vi "QWTB Algorithms Configurator Panel.vi"(8 "error in":errorcluster, 11 "session out":T1={"adc"={"niScope"={"channel cfg"=[], "sessions"=[], "multi cards"=FALSE, "channels"=0, "type"=enum."n/a", "memory [B/chn]"=0, "ext. clock [Hz]"=0.0, "samples count"=0, "use streaming"=FALSE, "proc setup"={"packet size [smpl]"=0, "current timeout [s]"=0.0, "blk2blk timeout [s]"=0.0, "event time"=timestamp(0 s since 1904-01-01), "temp sampl T [s]"=0.0, "data queue"=refnum, "stop notifier"=refnum, "proc ref"=refnum}, "sample width [B]"=0, "ranges [V]"=[], "trigger setup"={"coupling"=1, "level [V]"=0.0, "slope"=0, "mode"=enum."Immediate", "pre-trigger [%]"=0.0}, "fs [Hz]"=0.0, "bitres [bit]"=0, "clock source"=enum."VAL_NO_SOURCE"}, "3458A"={"channels"=[], "sync unit"={"VISA"="", "type"=enum."Picotest U6200A"}, "awg unit"={"type"=enum."Agilent 331xxA to 332xxA", "VISA"="", "enable 10MHz ref"=FALSE, "cmi ckd2"={"VISA"="", "clock source"=enum."Auto", "manual ref clk"=FALSE, "ref clock [Hz]"=0.0, "div mode"=enum."Set divisor directly"}, "cmi sync v3"={"VISA"="", "baud rate [bd/s]"=115200, "source"=enum."Auto", "hv range"=enum."1kV", "fsrc is fixed"=FALSE, "fsrc [Hz]"=10000000.0, "freq integ [s]"=1.0, "freq filter"=5, "trig level"=enum."TTL 5V", "chn1 mode"=enum."Source divider", "chn1 level"=enum."Positive 5V", "chn2 mode"=enum."Source divider", "chn2 level"=enum."Positive 5V", "chn2 div"=1, "chn3 mode"=enum."Chn 1 Active", "chn3 level"=enum."Positive 5V", "chn1 div entry"=enum."Calculate nearest divisor from measured fx", "chn1 dev limit [%]"=1.0, "chn1 check dev"=FALSE}, "trigger"={"source"=enum."Immediate", "slope"=enum."POS", "coupling"=enum."DC", "level [V]"=0.0, "hysteresis [V]"=0.0, "pre-trigger [%]"=0.0}, "HMF2500 cfg"={"Baud Rate"=9600, "Parity"=0, "Data Bits"=8, "Flow Control"=4}}, "sync mode"=enum."MASTER-SLAVE, MASTER clocked by TIMER", "streaming mode"=FALSE, "idn mode"=enum."Auto", "sampling mode"=enum."DCV", "sample memory [B]"=0, "proc setup"={"channel id"=0, "packet size [smpl]"=0, "current timeout [s]"=0.0, "blk2blk timeout [s]"=0.0, "event time"=timestamp(0 s since 1904-01-01), "stop notifier"=refnum, "data queues"=[], "proc refs"=[], "bus semaphore"=refnum}, "sample size [B]"=0, "sample count"=0, "aux data"={"channel id"=0, "valid?"=[], "gain [V]"=[], "timestamp [s]"=[], "Ts [s]"=0.0, "abs timestamp"=timestamp(0 s since 1904-01-01), "t [deg C]"=[], "multiplex timestamp [s]"=-1.0, "only multiplex?"=FALSE, "multiplex smpl offset"=0, "overflow?"=FALSE}, "ranges [V]"=[], "aperture [s]"=0.0, "LEVEL trigger"={"edge"=enum."POS", "level [V]"=0.0, "coupling"=enum."DC"}, "trigger mode"=enum."AUTO", "measure temp.?"=FALSE, "disp mesages"=[], "shared bus?"=FALSE, "disable display?"=FALSE, "aper mode"=enum."Manual", "aper rules"=[], "multiplex"={"cycles"=0, "delay [s]"=0.0, "enabled"=FALSE, "overhead [s]"=1.0, "tot smpls"=0, "sub-rec"=0, "overhead [%]"=0.0, "emulated"=FALSE}, "F8588 lpf"=enum."Off", "F8588 pll"=enum."Off", "F8588 couple"=enum."DC, auto", "fs"={"freq mode"=enum."fs or Ts", "fs [Hz]"=0.0, "fref [Hz]"=0.0, "mul"=0.0, "div"=0.0}, "fs mode"=enum."fs or Ts", "init timestamp"=timestamp(0 s since 1904-01-01), "last report timestamp"=timestamp(0 s since 1904-01-01)}, "dsdll"={"dsdll"={"dsdll path"=path "", "dsdll handle"=[], "output devices"=[], "capture devices"=[]}, "channels"=0, "device id"=0, "channel idns"=[], "proc setup"={"packet size [smpl]"=0, "current timeout [s]"=0.0, "blk2blk timeout [s]"=0.0, "event time"=timestamp(0 s since 1904-01-01), "data queue"=refnum, "stop notifier"=refnum, "proc ref"=refnum}, "samples count"=0, "fs [Hz]"=0.0}, "type"=enum."niScope", "channel idn str"=[], "aux instr idn str"=[], "modified?"=FALSE, "simadc"={"channels"=[], "range [V]"=0.0, "Ts step [s]"=0.0, "time [s]"=0.0, "fs [Hz]"=0.0, "count"=0, "smpl offset"=0, "set count"=0, "bit res"=0}, "force rst?"=FALSE, "exit mode"=enum."Immediate reset", "exit dly"=0.0, "exit tmr"=timestamp(0 s since 1904-01-01), "busy?"=FALSE, "accessed?"=FALSE, "multiplex"={"Type"=enum."Dummy", "gen com ssn"={"visa"="", "primary"=enum."None", "secondary"=enum."None", "channels"=[]}, "delay before [s]"=0.0, "delay post [s]"=0.0, "sequence"=[], "enabled"=FALSE, "ref timestamp [s]"=0.0, "idn string"="", "dev niScope"="", "niScope idx"=0, "QPMX ssn"={"visa"="", "switch mode"=enum."Switched by TWM", "sequence"=[], "timing delays"=[], "polarity"=enum."Positive", "ss delay (s)"=2.0, "internal timer (s)"=1.0, "Last loaded sequence file"=path "", "startup delay (s)"=2.0}, "VISA mux ssn"={"VISA"="", "paths"=[], "idn command"="", "serial cfg"={"Baud rate"=9600, "Data bits"=8, "Parity"=0, "Stop bits"=10, "Flow control"=0, "End Mode Read"=enum."None", "End Mode Write"=enum."None", "Term character"=0, "Term enable"=FALSE}}}, "keysight dso"={"VISA"="", "channels"=[], "bw limit [Hz]"=0.0, "resolution"=enum."Basic", "trig noise reject"=enum."Normal", "N"=0, "trigger config"={"trigger source"=enum."Immediate", "trigger slope"=enum."Negative", "level [V]"=0.0, "hysteresis [V]"=0.001, "pre-trig [%]"=50}, "fs [Hz]"=0.0, "timeout stop"=timestamp(0 s since 1904-01-01), "waiting for opc"=FALSE, "fetch offset [smpl]"=0, "abs timestamp"=timestamp(0 s since 1904-01-01), "ranges [V]"=[], "decimation"=1.0, "ext ref"=FALSE, "emulate aperture"=FALSE, "model"=enum."DSO91304"}, "cdaq"={"mclk [Hz]"=12800000.0, "ADC task"="", "mclk reference"="", "fs [Hz]"=50000.0, "queue adc cmd"=refnum, "queue adc data"=refnum, "adc proc ref"=refnum, "channels"=[], "last channels"=[], "timeout"=timestamp(0 s since 1904-01-01), "N"=1000, "mclk mode"=enum."Free running", "ext mclk source"=""}, "ignore overload"=FALSE, "ADS127L21"={"VISA"="", "chn list"=[], "record size"=0, "phys. channels"=0, "adc fifo size"=0, "channels"=[], "ext refclk?"=FALSE, "fs [Hz]"=0.0, "ext refclk [Hz]"=0.0, "meas refclk [Hz]"=0.0, "EXTOUT mode"=enum."ADCCLK", "EXTOUT polarity"=enum."NORM", "EXTOUT divisor"=0}}, "sequence"=[], "sequence setup"={"group setups"=[], "rec count"=0, "range mode"=enum."Keep defaults", "fs mode"=enum."Frequency", "rng even"=0.0, "rng odd"=0.0, "folder"=path "", "name base"="", "meas id"=0, "settle [s]"=0.0, "comment"="", "avg count"=0, "fs-abs-fr fr"=0.0, "fs-abs-fr fs"=0.0, "fs-div fr"=0.0, "fs-div div"=0.0, "fs-mn fr"=0.0, "fs-mn mul"=0.0, "fs-mn div"=0.0, "fs-rat fr"=0.0, "fs-rat rat"=0.0}, "golpi"=refnum, "processing setup"={"mode"=enum."Raw", "call after avgs?"=FALSE, "calculate?"=FALSE, "raw mode"={"command"="", "result mode"=enum."Display console output (only Octave)", "res variable"=""}, "QWTB"={"QWTB path"=path "F:/TWM/octprog/qwtb", "alg filter path"="octprog\\qwtb_list.info", "alg ids"=[], "alg parameters"=[], "parsed parameters"=[], "selected alg id"="", "selected unc mode"=enum."None", "qwtb mcc"=100, "qwtb timeout"=90, "qwtb covg"=95.0, "qwtb ofs"=0, "qwtb lim data"=0, "multicore"={"jobs folder"=path "", "cores"=0, "max jobs"=0, "mode"=enum."Singlecore"}, "unc once?"=FALSE, "qwtb tstemp"=enum."Enabled (default)", "octave reset"=FALSE, "exec mode"=enum."Single-core"}}, "corrections"={"transducers"={"channels"=[], "last path"=path "", "root path"=path ""}, "digitizer"={"last path"=path "", "channel paths"=[], "channel idns"=[], "correction name"="", "channel names"=[], "folders to copy"=[], "channel valid"=[], "correction path"=path "", "correction rel path"="", "rel folders to copy"=[], "root path"=path ""}}, "assist cfg"={"P"=0, "Q"=0, "rel shift"=0.0, "ref freq"=0.0, "min fs"=0.0, "max fs tol"=0.0, "min int"=0.0, "max int"=0.0, "max err"=0.0, "max timeout"=0.0}} {"corrections"."transducers"."channels"."Phase index" min=1 step=1; "adc"."ADS127L21"."channels"."Channel" min=1 max=8 step=1; "adc"."ADS127L21"."channels"."Range [Vpk]" items=["±1.65V", "±2V"]; "adc"."cdaq"."last channels"."Channel id" min=0 step=1; "adc"."cdaq"."channels"."Channel id" min=0 step=1; "adc"."keysight dso"."decimation" min=1.0; "adc"."keysight dso"."bw limit [Hz]" format="%#_6p"; "adc"."keysight dso"."channels"."Offset [V]" format="%#_6p"; "adc"."keysight dso"."channels"."Range [Vpk]" min=0.0 format="%#_6p"; "adc"."keysight dso"."channels"."Channel" min=1; "adc"."multiplex"."VISA mux ssn"."serial cfg"."Flow control" items=["None", "XON/XOFF", "CTS/RTS", "XON/XOFF + CTS/RTS", "DTR/DSR", "XON/XOFF + DTR/DSR"]; "adc"."multiplex"."VISA mux ssn"."serial cfg"."Stop bits" items=["1 bit"=10, "1.5 bits"=15, "2 bits"=20]; "adc"."multiplex"."VISA mux ssn"."serial cfg"."Parity" items=["None", "Odd", "Even", "Mark", "Space"]; "adc"."multiplex"."VISA mux ssn"."serial cfg"."Data bits" items=["5 bits"=5, "6 bits"=6, "7 bits"=7, "8 bits"=8]; "adc"."multiplex"."VISA mux ssn"."serial cfg"."Baud rate" items=["150 Bd"=150, "300 Bd"=300, "600 Bd"=600, "1200 Bd"=1200, "2400 Bd"=2400, "4800 Bd"=4800, "9600 Bd"=9600, "19.2 kBd"=19200, "38.4 kBd"=38400, "57.6 kBd"=57600, "115.2 kBd"=115200]; "adc"."multiplex"."QPMX ssn"."startup delay (s)" min=0.0 step=1.0; "adc"."multiplex"."QPMX ssn"."internal timer (s)" min=0.0 step=1.0; "adc"."multiplex"."QPMX ssn"."ss delay (s)" min=0.0 step=1.0; "adc"."multiplex"."QPMX ssn"."timing delays" min=1 max=255 step=1; "adc"."3458A"."awg unit"."HMF2500 cfg"."Flow Control" items=["None", "XON/XOFF", "RTS/CTS", "XON/XOFF & RTS/CTS", "DTR/DSR", "XON/XOFF & DTR/DSR"]; "adc"."3458A"."awg unit"."HMF2500 cfg"."Data Bits" items=["7"=7, "8"=8]; "adc"."3458A"."awg unit"."HMF2500 cfg"."Parity" items=["None", "Odd", "Even", "Mark", "Space"]; "adc"."3458A"."awg unit"."HMF2500 cfg"."Baud Rate" items=["300"=300, "600"=600, "1200"=1200, "2400"=2400, "4800"=4800, "9600"=9600, "19200"=19200]; "adc"."3458A"."awg unit"."cmi sync v3"."chn2 div" min=1 max=100000000 step=1; "adc"."3458A"."awg unit"."cmi sync v3"."fsrc [Hz]" format="%_8p"; "adc"."3458A"."channels"."Range [Vpk]" min=0.0; "adc"."niScope"."trigger setup"."pre-trigger [%]" format="%.2f"; "adc"."niScope"."trigger setup"."level [V]" format="%.2f"; "adc"."niScope"."trigger setup"."coupling" items=["AC"=0, "DC"=1, "HF Reject"=3, "LF Reject"=4, "AC Plus HF Reject"=1001]; "adc"."niScope"."channel cfg"."Range [Vpk]" min=0.0; "adc"."niScope"."channel cfg"."Channel" min=0}) -> (0 "error out":errorcluster)   [LabVIEW 2020]
doc: "Configuration panel for QWTB algorithms."
uses:
  Meas Session.ctl
  adc/ADC Session.ctl
  drivers/niScope/niScope Session.ctl
  drivers/niScope/niScope Virtual Channel Config.ctl
  drivers/niScope/niScope Virtual Channel Mode.ctl
  drivers/niScope/niScope Virtual Channel Input Z.ctl
  drivers/niScope/niScope Virtual Channel Coupling.ctl
  drivers/niScope/niScope Type.ctl
  drivers/niScope/niScope Digitizing Process Options.ctl
  drivers/niScope/niScope Data Packet.ctl
  drivers/niScope/niScope Trigger Setup.ctl
  <instrlib>/niScope/Controls/niScope trigger coupling.ctl
  <instrlib>/niScope/Controls/niScope trigger slope.ctl
  drivers/niScope/niScope Reference Clock.ctl
  drivers/DMM/3458A Digitizer Session.ctl
  drivers/DMM/3458A Virtual Channel Config.ctl
  drivers/Counter/Counter Session.ctl
  drivers/Counter/Counter Type.ctl
  drivers/AWG/AWG Session.ctl
  drivers/AWG/AWG Type.ctl
  drivers/AWG/CMI Clock Divider v2/CMI ckd2 Session.ctl
  drivers/AWG/CMI Clock Divider v2/CMI ckd2 Source Mode.ctl
  drivers/AWG/CMI Clock Divider v2/CMI ckd2 Divisor Mode.ctl
  drivers/AWG/CMI Sync V3/CMI Sync V3 session.ctl
  drivers/AWG/CMI Sync V3/Configure/CMI Sync V3 Reference Clock Source.ctl
  drivers/AWG/CMI Sync V3/Configure/CMI Sync V3 HV input Range.ctl
  drivers/AWG/CMI Sync V3/Configure/CMI Sync V3 Trigger Input Level.ctl
  drivers/AWG/CMI Sync V3/Configure/CMI Sync V3 Channel 1 Mode.ctl
  drivers/AWG/CMI Sync V3/Configure/CMI Sync V3 Channel Output Levels.ctl
  drivers/AWG/CMI Sync V3/Configure/CMI Sync V3 Channel 2 Mode.ctl
  drivers/AWG/CMI Sync V3/Configure/CMI Sync V3 Channel 3 Mode.ctl
  drivers/AWG/CMI Sync V3/Configure/CMI Sync V3 Channel 1 Divisor Entry Mode.ctl
  adc/ADC Trig Config.ctl
  adc/ADC Trig Mode Source.ctl
  adc/ADC Trig Slope.ctl
  adc/ADC Trig Coupling.ctl
  drivers/AWG/RaS HMF2500/HMF2500 Config.ctl
  drivers/DMM/3458A Sync Mode.ctl
  drivers/DMM/3458A Idn Mode.ctl
  drivers/DMM/3458A Digitizing Low Levels/Configure/Sampling Mode.ctl
  drivers/DMM/3458A Digitizing Process Options.ctl
  drivers/DMM/3458A Data Packet.ctl
  drivers/DMM/3458A Aux Record Data.ctl
  drivers/DMM/3458A Digitizing Low Levels/Configure/Level Setup.ctl
  drivers/DMM/3458A Digitizing Low Levels/Configure/First Sample Trigger.ctl
  drivers/DMM/3458A Aperture Selection Mode.ctl
  drivers/DMM/3458A Multiplexing Config.ctl
  drivers/Fluke 8588A/F8588A Low Pass Filter.ctl
  drivers/Fluke 8588A/F8588A Phase Lock.ctl
  drivers/Fluke 8588A/F8588A Coupling.ctl
  drivers/DMM/3458A Sampling Rate.ctl
  drivers/AWG/AWG Clock Setup Mode.ctl
  drivers/DMM/3458A Sample Rate Mode.ctl
  drivers/dsdll/DSDLL Session.ctl
  drivers/dsdll/dsdll/dsdll_instance.ctl
  drivers/dsdll/dsdll/dsdll_device_record.ctl
  drivers/dsdll/DSDLL Process Config.ctl
  drivers/dsdll/DSDLL Data Packet.ctl
  adc/ADC Type.ctl
  drivers/simulated_adc/SimAdc Config.ctl
  drivers/simulated_adc/SimAdc Channel Cfg.ctl
  adc/ADC On Close Action.ctl
  adc/Multiplexer/MPX Session.ctl
  adc/Multiplexer/MPX Type.ctl
  drivers/Multiplexers/Generic COM/GCOMM Session.ctl
  drivers/Multiplexers/Generic COM/GCOMM Signal.ctl
  drivers/Multiplexers/Generic COM/GCOMM Virtual Channel.ctl
  drivers/Multiplexers/Generic COM/GCOMM Logic State.ctl
  drivers/Multiplexers/Generic COM/QPMX Session.ctl
  drivers/Multiplexers/QPMX/QPMX switch mode.ctl
  drivers/Multiplexers/QPMX/QPMX polarity.ctl
  drivers/Multiplexers/Generic VISA commands/GVISA Mux Session.ctl
  drivers/Multiplexers/Generic VISA commands/GVISA Mux Path Entry.ctl
  drivers/Multiplexers/Generic VISA commands/met_serial_setup.ctl
  drivers/Agilent DSO 90000/Virtual Digitizer/KeDSO session.ctl
  drivers/Agilent DSO 90000/Virtual Digitizer/KeDSO Virtual Channel.ctl
  drivers/Agilent DSO 90000/Virtual Digitizer/KeDSO High Resolution Mode.ctl
  drivers/Agilent DSO 90000/Virtual Digitizer/KeDSO Trigger Setup.ctl
  drivers/Agilent DSO 90000/Virtual Digitizer/KeDSO Trigger Source.ctl
  drivers/Agilent DSO 90000/Public/Utility/DSO type.ctl
  drivers/cdaq/cDAQ Session.ctl
  drivers/cdaq/low_level_old/cdaq_anal_adc_command.ctl
  drivers/cdaq/low_level_old/cdaq_anal_adc_data.ctl
  drivers/cdaq/cDAQ Virtual Channel.ctl
  drivers/cdaq/cDAQ Master Clock Mode.ctl
  drivers/CMI_ADS127L21/CMI ADS127L21 - Session.ctl
  drivers/CMI_ADS127L21/CMI ADS127L21 - Record Channel.ctl
  drivers/CMI_ADS127L21/CMI ADS127L21 - Input Range.ctl
  drivers/CMI_ADS127L21/CMI ADS127L21 - Input Mode.ctl
  drivers/CMI_ADS127L21/CMI ADS127L21 - Input Impedance.ctl
  drivers/CMI_ADS127L21/CMI ADS127L21 - EXTOUT Mode.ctl
  drivers/CMI_ADS127L21/CMI ADS127L21 - EXTOUT Polarity.ctl
  Meas Sequence Item.ctl
  Meas Sampling Configuration.ctl
  Meas Proc QWTB Algorithm Parameter Data.ctl
  Meas Sequence Configuration.ctl
  Meas Range Mode.ctl
  Meas Sampling Rate Mode.ctl
  octave/golpi/mpc/golpi_session_ref.ctl
  octave/golpi/mpc/golpi_session.ctl
  octave/golpi/GOLPI reference Type Def.ctl
  octave/golpi/Pipe Handle.ctl
  Meas Process Config.ctl
  Meas Process Mode.ctl
  Meas Process Raw Config.ctl
  Meas Process Raw Result Mode.ctl
  Meas Proc QWTB Setup.ctl
  Meas Proc QWTB Uncertainty Mode.ctl
  Meas Proc QWTB Multicore Setup.ctl
  Meas Proc QWTB Multicore Type.ctl
  Meas Process Time Stamp Mode.ctl
  Meas Proc QWTB Exec Mode.ctl
  Corrections/Corr Setup.ctl
  Corrections/Corr Tranducer Item.ctl
  Corrections/Corr Digitizers.ctl
  Assist/Assist Panel Setup.ctl
  octave/infolib/infolib.lvlib
  drivers/niScope/niScope Virtual Digitizer.lvlib
  drivers/DMM/3458A Virtual Digitizer.lvlib
  drivers/Counter/Counter.lvlib
  drivers/AWG/AWG.lvlib
  drivers/AWG/CMI Sync V3/CMI Sync Unit V3.lvlib
  drivers/DMM/3458A Digitizing Low Levels/3458A Digitizing Low Levels.lvlib
  drivers/dsdll/dsdll/dsdll.lvlib
  drivers/dsdll/DSDLL Virtual Digitizer.lvlib
  drivers/Agilent DSO 90000/Agilent 90000 Series.lvlib
  octave/golpi/LV Process library.lvlib
  octave/golpi/GOLPI library.lvlib
  octave/golpi/mpc/GOLPI Multi Process.lvlib
panel:
  in  "btn help":bool
  out "alg filter path":path caption="TWM algorithms filter path"
  in  "btn scan algs":bool
  in  "btn load all algs":bool
  in  "btn load alg cfg":bool
  out "qwtb path":path caption="QWTB instance path"
  in  "btn rem":bool
  in  "btn add":bool
  in  "list listed":i32(listbox) caption="Listed TWM algorithms"
  in  "list available":i32(listbox) caption="Found TWM algorithms"
  in  "btn save":bool
  in  "btn ok":bool
  in  "info":string caption="qwtb_list.info (editable)"
  # "TWM will only display QWTB algorithms that are listed in matrix 'list of supported algorithms'. \nEach algorithm can have optional section that defines quantities display formats in TWM, graphs, quantity types, etc.\nYou can edit 'qwtb_list.info' file manually or you can use menus below. You can also reload default algorithm configurations from algorithms folder (from file 'alg_twm.info' in algorithm folder if present)."
  # "ADC:"
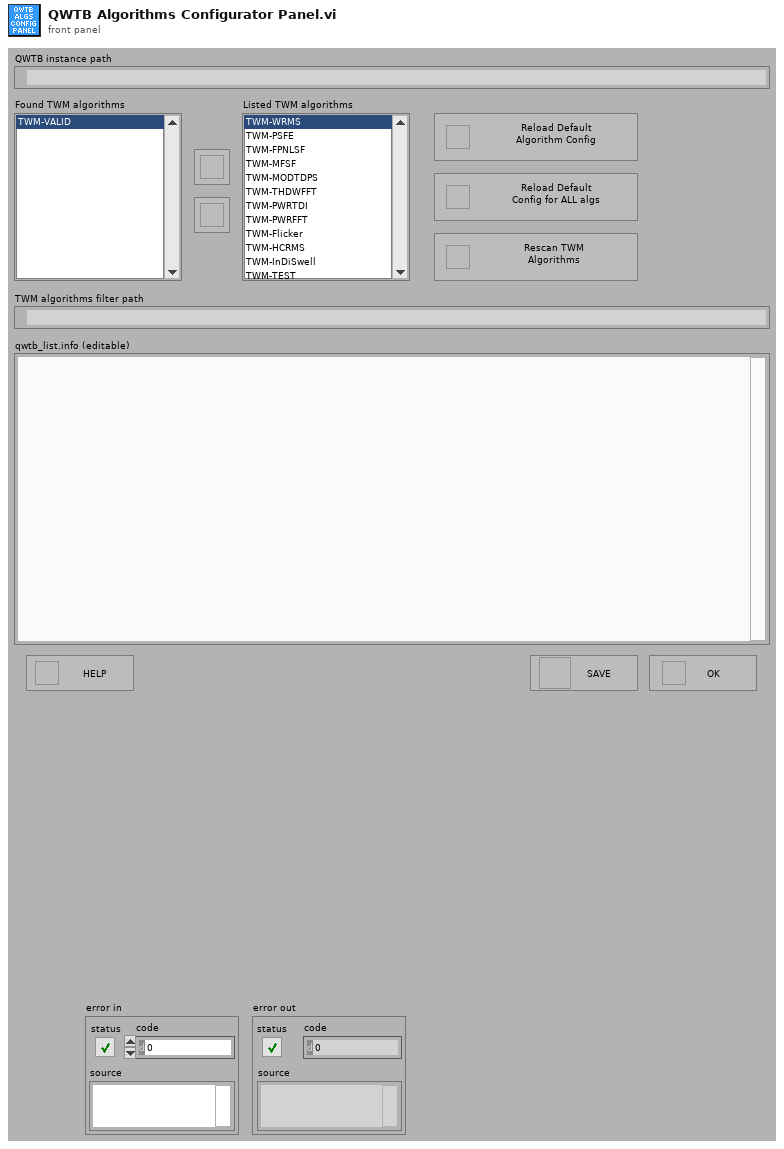
[diagram p1: front panel]
types:
  T1 = typedef "Meas Session.ctl" = cluster{"adc":T2, "sequence":T89[], "sequence setup":T92, "golpi":T95, "processing setup":T96, "corrections":T106, "assist cfg":T109}
  T2 = typedef "ADC Session.ctl" = cluster{"niScope":T3, "3458A":T14, "dsdll":T53, "type":T57, "channel idn str":string[], "aux instr idn str":string[], "modified?":bool, "simadc":T58, "force rst?":bool, "exit mode":T60, "exit dly":dbl, "exit tmr":timestamp, "busy?":bool, "accessed?":bool, "multiplex":T61, "keysight dso":T73, "cdaq":T79, "ignore overload":bool, "ADS127L21":T82}
  T3 = typedef "niScope Virtual Digitizer.lvlib/niScope Session.ctl" = cluster{"channel cfg":T4[], "sessions":refnum<k20>[], "multi cards":bool, "channels":i32, "type":T8, "memory [B/chn]":i32, "ext. clock [Hz]":dbl, "samples count":i64, "use streaming":bool, "proc setup":T9, "sample width [B]":i32, "ranges [V]":dbl[], "trigger setup":T10, "fs [Hz]":dbl, "bitres [bit]":i32, "clock source":T13}
  T4 = typedef "niScope Virtual Digitizer.lvlib/niScope Virtual Channel Config.ctl" = cluster{"Address":refnum<k15>, "Channel":i32, "Mode":T5, "Input Z":T6, "Coupling":T7, "Range [Vpk]":dbl, "btn clr":bool, "btn up":bool, "btn down":bool}
  T5 = typedef "niScope Virtual Digitizer.lvlib/niScope Virtual Channel Mode.ctl" = enum16{"Single ended", "Unbal. differential", "Differential"}
  T6 = typedef "niScope Virtual Digitizer.lvlib/niScope Virtual Channel Input Z.ctl" = enum16{"1 MOhm", "50 Ohm"}
  T7 = typedef "niScope Virtual Digitizer.lvlib/niScope Virtual Channel Coupling.ctl" = enum16{"AC", "DC", "GND"}
  T8 = typedef "niScope Virtual Digitizer.lvlib/niScope Type.ctl" = enum16{"n/a", "5922"}
  T9 = typedef "niScope Virtual Digitizer.lvlib/niScope Digitizing Process Options.ctl" = cluster{"packet size [smpl]":i64, "current timeout [s]":dbl, "blk2blk timeout [s]":dbl, "event time":timestamp, "temp sampl T [s]":dbl, "data queue":refnum<queue>, "stop notifier":refnum<notifier>, "proc ref":refnum<vi>}
  T10 = typedef "niScope Virtual Digitizer.lvlib/niScope Trigger Setup.ctl" = cluster{"coupling":T11, "level [V]":dbl, "slope":T12, "mode":enum16{"Immediate", "External", "Level"}, "pre-trigger [%]":dbl}
  T11 = typedef "niScope trigger coupling.ctl" = u16
  T12 = typedef "niScope trigger slope.ctl" = i32
  T13 = typedef "niScope Virtual Digitizer.lvlib/niScope Reference Clock.ctl" = enum16{"VAL_NO_SOURCE", "VAL_CLK_IN", "VAL_PXI_CLOCK", "VAL_EXTERNAL"}
  T14 = typedef "3458A Virtual Digitizer.lvlib/3458A Digitizer Session.ctl" = cluster{"channels":T15[], "sync unit":T16, "awg unit":T18, "sync mode":T37, "streaming mode":bool, "idn mode":T38, "sampling mode":T39, "sample memory [B]":i32, "proc setup":T40, "sample size [B]":i32, "sample count":i32, "aux data":T42, "ranges [V]":dbl[], "aperture [s]":dbl, "LEVEL trigger":T43, "trigger mode":T44, "measure temp.?":bool, "disp mesages":string[], "shared bus?":bool, "disable display?":bool, "aper mode":T45, "aper rules":dbl[][], "multiplex":T46, "F8588 lpf":T47, "F8588 pll":T48, "F8588 couple":T49, "fs":T50, "fs mode":T52, "init timestamp":timestamp, "last report timestamp":timestamp}
  T15 = typedef "3458A Virtual Digitizer.lvlib/3458A Virtual Channel Config.ctl" = cluster{"VISA":refnum<visa-resource-name>, "Range [Vpk]":dbl, "btn clr":bool, "btn up":bool, "btn down":bool, "F8588":bool, "F8588 guard":bool}
  T16 = typedef "Counter.lvlib/Counter Session.ctl" = cluster{"VISA":refnum<visa-resource-name>, "type":T17}
  T17 = typedef "Counter.lvlib/Counter Type.ctl" = enum16{"Picotest U6200A", "dummy"}
  T18 = typedef "AWG.lvlib/AWG Session.ctl" = cluster{"type":T19, "VISA":refnum<visa-resource-name>, "enable 10MHz ref":bool, "cmi ckd2":T20, "cmi sync v3":T23, "trigger":T32, "HMF2500 cfg":T36}
  T19 = typedef "AWG.lvlib/AWG Type.ctl" = enum16{"Agilent 331xxA to 332xxA", "Agilent 335xxA to 336xxA", "Tektronix AFG3101C", "R&S HMF25xx", "CMI Clock Divider v2", "CMI Sync Unit V3", "dummy"}
  T20 = typedef "AWG.lvlib/CMI ckd2 Session.ctl" = cluster{"VISA":refnum<visa-resource-name>, "clock source":T21, "manual ref clk":bool, "ref clock [Hz]":dbl, "div mode":T22}
  T21 = typedef "AWG.lvlib/CMI ckd2 Source Mode.ctl" = enum16{"Auto", "LF clock", "HF clock", "Internal"}
  T22 = typedef "AWG.lvlib/CMI ckd2 Divisor Mode.ctl" = enum16{"Set divisor directly", "Set divisor by frequency"}
  T23 = typedef "AWG.lvlib/CMI Sync Unit V3.lvlib/CMI Sync V3 session.ctl" = cluster{"VISA":refnum<visa-resource-name>, "baud rate [bd/s]":i32, "source":T24, "hv range":T25, "fsrc is fixed":bool, "fsrc [Hz]":dbl, "freq integ [s]":dbl, "freq filter":i32, "trig level":T26, "chn1 mode":T27, "chn1 level":T28, "chn2 mode":T29, "chn2 level":T28, "chn2 div":i32, "chn3 mode":T30, "chn3 level":T28, "chn1 div entry":T31, "chn1 dev limit [%]":dbl, "chn1 check dev":bool}
  T24 = typedef "AWG.lvlib/CMI Sync Unit V3.lvlib/CMI Sync V3 Reference Clock Source.ctl" = enum16{"Auto", "Internal", "Logic", "Sine", "HV"}
  T25 = typedef "AWG.lvlib/CMI Sync Unit V3.lvlib/CMI Sync V3 HV input Range.ctl" = enum16{"10V", "60V", "250V", "1kV"}
  T26 = typedef "AWG.lvlib/CMI Sync Unit V3.lvlib/CMI Sync V3 Trigger Input Level.ctl" = enum16{"LVCMOS 3V3", "TTL 5V"}
  T27 = typedef "AWG.lvlib/CMI Sync Unit V3.lvlib/CMI Sync V3 Channel 1 Mode.ctl" = enum16{"Source divider", "DDS absolute", "DDS ratio", "DDS ratio M/N"}
  T28 = typedef "AWG.lvlib/CMI Sync Unit V3.lvlib/CMI Sync V3 Channel Output Levels.ctl" = enum16{"Positive 3V3", "Negative 3V3", "Positive 5V", "Negative 5V"}
  T29 = typedef "AWG.lvlib/CMI Sync Unit V3.lvlib/CMI Sync V3 Channel 2 Mode.ctl" = enum16{"Source divider", "Chn 1 divide"}
  T30 = typedef "AWG.lvlib/CMI Sync Unit V3.lvlib/CMI Sync V3 Channel 3 Mode.ctl" = enum16{"Chn 1 Active", "Chn 2 Active", "Chn 1 Trigger", "Chn 2 Trigger", "Gate", "PPS", "10MHz"}
  T31 = typedef "AWG.lvlib/CMI Sync Unit V3.lvlib/CMI Sync V3 Channel 1 Divisor Entry Mode.ctl" = enum16{"Set divisor directly", "Calculate nearest divisor from measured fx"}
  T32 = typedef "ADC Trig Config.ctl" = cluster{"source":T33, "slope":T34, "coupling":T35, "level [V]":dbl, "hysteresis [V]":dbl, "pre-trigger [%]":dbl}
  T33 = typedef "ADC Trig Mode Source.ctl" = enum16{"Immediate", "External", "Level"}
  T34 = typedef "ADC Trig Slope.ctl" = enum16{"POS", "NEG"}
  T35 = typedef "ADC Trig Coupling.ctl" = enum16{"DC", "AC"}
  T36 = typedef "AWG.lvlib/HMF2500 Config.ctl" = cluster{"Baud Rate":u32, "Parity":u16, "Data Bits":u16, "Flow Control":u16}
  T37 = typedef "3458A Virtual Digitizer.lvlib/3458A Sync Mode.ctl" = enum16{"MASTER-SLAVE, MASTER clocked by TIMER", "MASTER-SLAVE, MASTER clocked by AWG", "ALL clocked by AWG", "MASTER-SLAVE, ALL clocked by TIMER", "ALL clocked by AWG with DFLL"}
  T38 = typedef "3458A Virtual Digitizer.lvlib/3458A Idn Mode.ctl" = enum16{"Auto", "Sequential (chn A, chn B, ...)", "From calibration string"}
  T39 = typedef "3458A Virtual Digitizer.lvlib/3458A Digitizing Low Levels.lvlib/Sampling Mode.ctl" = enum16{"DCV", "DSDC", "DSAC"}
  T40 = typedef "3458A Virtual Digitizer.lvlib/3458A Digitizing Process Options.ctl" = cluster{"channel id":i32, "packet size [smpl]":i32, "current timeout [s]":dbl, "blk2blk timeout [s]":dbl, "event time":timestamp, "stop notifier":refnum<notifier>, "data queues":refnum<queue>[], "proc refs":refnum<vi>[], "bus semaphore":T41}
  T41 = typedef "Semaphore RefNum" = refnum<k1>
  T42 = typedef "3458A Virtual Digitizer.lvlib/3458A Aux Record Data.ctl" = cluster{"channel id":i32, "valid?":bool[], "gain [V]":dbl[], "timestamp [s]":dbl[], "Ts [s]":dbl, "abs timestamp":timestamp, "t [deg C]":dbl[], "multiplex timestamp [s]":dbl, "only multiplex?":bool, "multiplex smpl offset":i64, "overflow?":bool}
  T43 = typedef "3458A Virtual Digitizer.lvlib/3458A Digitizing Low Levels.lvlib/Level Setup.ctl" = cluster{"edge":enum16{"POS", "NEG"}, "level [V]":dbl, "coupling":enum16{"DC", "AC"}}
  T44 = typedef "3458A Virtual Digitizer.lvlib/3458A Digitizing Low Levels.lvlib/First Sample Trigger.ctl" = enum16{"AUTO", "EXT", "SYN", "SGL", "HOLD", "LEVEL"}
  T45 = typedef "3458A Virtual Digitizer.lvlib/3458A Aperture Selection Mode.ctl" = enum16{"Manual", "Maximum", "Table"}
  T46 = typedef "3458A Virtual Digitizer.lvlib/3458A Multiplexing Config.ctl" = cluster{"cycles":i32, "delay [s]":dbl, "enabled":bool, "overhead [s]":dbl, "tot smpls":i64, "sub-rec":i32, "overhead [%]":dbl, "emulated":bool}
  T47 = typedef "F8588A Low Pass Filter.ctl" = enum16{"Off", "100 kHz", "3 MHz"}
  T48 = typedef "F8588A Phase Lock.ctl" = enum16{"Off", "1 MHz", "10 MHz"}
  T49 = typedef "F8588A Coupling.ctl" = enum16{"AC, 1 MOhm", "AC, 10 MOhm", "DC, 1 MOhm", "DC, 10 MOhm", "DC, auto"}
  T50 = typedef "3458A Virtual Digitizer.lvlib/3458A Sampling Rate.ctl" = cluster{"freq mode":T51, "fs [Hz]":dbl, "fref [Hz]":dbl, "mul":dbl, "div":dbl}
  T51 = typedef "AWG.lvlib/AWG Clock Setup Mode.ctl" = enum16{"fs or Ts", "fs or Ts with fref", "fref/N", "fref*M/N", "fref*Ratio"}
  T52 = typedef "3458A Sample Rate Mode.ctl" = enum16{"fs or Ts", "fs*M/N"}
  T53 = typedef "DSDLL Virtual Digitizer.lvlib/DSDLL Session.ctl" = cluster{"dsdll":T54, "channels":i32, "device id":i32, "channel idns":string[], "proc setup":T56, "samples count":i32, "fs [Hz]":dbl}
  T54 = typedef "dsdll.lvlib/dsdll_instance.ctl" = cluster{"dsdll path":path, "dsdll handle":u8[], "output devices":T55[], "capture devices":T55[]}
  T55 = typedef "dsdll.lvlib/dsdll_device_record.ctl" = cluster{"guid":u8[], "name":string}
  T56 = typedef "DSDLL Virtual Digitizer.lvlib/DSDLL Process Config.ctl" = cluster{"packet size [smpl]":i32, "current timeout [s]":dbl, "blk2blk timeout [s]":dbl, "event time":timestamp, "data queue":refnum<queue>, "stop notifier":refnum<notifier>, "proc ref":refnum<vi>}
  T57 = typedef "ADC Type.ctl" = enum16{"niScope", "3458A", "DirectSound DLL", "Keysight DSO", "cDAQ ADC", "CMI ADS127L21", "dummy"}
  T58 = typedef "SimAdc Config.ctl" = cluster{"channels":T59[], "range [V]":dbl, "Ts step [s]":dbl, "time [s]":dbl, "fs [Hz]":dbl, "count":i64, "smpl offset":i64, "set count":i64, "bit res":i32}
  T59 = typedef "SimAdc Channel Cfg.ctl" = cluster{"harmonics":dbl[][], "btn clear":bool, "noise":dbl, "fundamental [Hz]":dbl}
  T60 = typedef "ADC On Close Action.ctl" = enum16{"Immediate reset", "Delayed reset"}
  T61 = typedef "MPX Session.ctl" = cluster{"Type":T62, "gen com ssn":T63, "delay before [s]":dbl, "delay post [s]":dbl, "sequence":string[], "enabled":bool, "ref timestamp [s]":dbl, "idn string":string, "dev niScope":refnum<k15>, "niScope idx":i32, "QPMX ssn":T67, "VISA mux ssn":T70}
  T62 = typedef "MPX Type.ctl" = enum16{"Dummy", "Generic - COM port", "Generic - niScope PFI", "Generic - VISA commands", "QPMX"}
  T63 = typedef "GCOMM Session.ctl" = cluster{"visa":refnum<visa-resource-name>, "primary":T64, "secondary":T64, "channels":T65[]}
  T64 = typedef "GCOMM Signal.ctl" = enum16{"None", "DTR", "RTS"}
  T65 = typedef "GCOMM Virtual Channel.ctl" = cluster{"Primary:":T66, "Secondary:":T66, "btn clr":bool, "btn up":bool, "btn down":bool, "Tag:":string}
  T66 = typedef "GCOMM Logic State.ctl" = enum16{"OFF", "ON"}
  T67 = typedef "QPMX Session.ctl" = cluster{"visa":refnum<visa-resource-name>, "switch mode":T68, "sequence":bool[][], "timing delays":u32[], "polarity":T69, "ss delay (s)":dbl, "internal timer (s)":dbl, "Last loaded sequence file":path, "startup delay (s)":dbl}
  T68 = typedef "QPMX switch mode.ctl" = enum16{"Switched by TWM", "Switched by external clock", "Switched by internal clock"}
  T69 = typedef "QPMX polarity.ctl" = enum16{"Positive", "Negative"}
  T70 = typedef "GVISA Mux Session.ctl" = cluster{"VISA":refnum<visa-resource-name>, "paths":T71[], "idn command":string, "serial cfg":T72}
  T71 = typedef "GVISA Mux Path Entry.ctl" = cluster{"Tag:":string, "Command:":string, "btn clr":bool, "btn up":bool, "btn down":bool}
  T72 = typedef "met_serial_setup.ctl" = cluster{"Baud rate":i32, "Data bits":i32, "Parity":i32, "Stop bits":i32, "Flow control":i32, "End Mode Read":enum16{"None", "Last Bit", "TermChar"}, "End Mode Write":enum16{"None", "Last Bit", "TermChar"}, "Term character":u8, "Term enable":bool}
  T73 = typedef "KeDSO session.ctl" = cluster{"VISA":refnum<visa-resource-name>, "channels":T74[], "bw limit [Hz]":dbl, "resolution":T75, "trig noise reject":enum16{"Normal", "High Sensitivity"}, "N":i64, "trigger config":T76, "fs [Hz]":dbl, "timeout stop":timestamp, "waiting for opc":bool, "fetch offset [smpl]":i64, "abs timestamp":timestamp, "ranges [V]":dbl[], "decimation":dbl, "ext ref":bool, "emulate aperture":bool, "model":T78}
  T74 = typedef "KeDSO Virtual Channel.ctl" = cluster{"Channel":i32, "Range [Vpk]":dbl, "btn clr":bool, "btn up":bool, "btn down":bool, "Offset [V]":dbl, "Coupling":enum16{"DC", "DC50", "AC", "LFR1"}, "bw limit enab":bool}
  T75 = typedef "KeDSO High Resolution Mode.ctl" = enum16{"Basic", "High-res AUTO", "Min. 9-bits", "Min. 10-bits", "Min. 11-bits", "Min. 12-bits", "Fixed 11-bits", "Fixed 12-bits", "Fixed 13-bits", "Fixed 14-bits", "Fixed 15-bits", "Fixed 16-bits"}
  T76 = typedef "KeDSO Trigger Setup.ctl" = cluster{"trigger source":T77, "trigger slope":enum16{"Negative", "Positive", "Either"}, "level [V]":dbl, "hysteresis [V]":dbl, "pre-trig [%]":i32}
  T77 = typedef "KeDSO Trigger Source.ctl" = enum16{"Immediate", "Level", "AUX"}
  T78 = typedef "Agilent 90000 Series.lvlib/DSO type.ctl" = enum16{"DSO91304", "DSO91204", "DSO90804", "DSO90604", "DSO90404", "DSO90254", "DSA91304", "DSA91204", "DSA90804", "DSA90604", "DSA90404", "DSA90254", "DSO9104", "DSO9254", "DSO9404", "MSO9104", "MSO9254", "MSO9404", "MSO9064", "DSO9064", "DSOX91604", "DSOX92004", "DSOX92504", "DSOX92804", "DSOX93204", "DSO93004", "DSO9024H", "DSO9054H", "DSO9104H", "DSO9204H", "DSOS054A", "DSOS104A", "DSOS204A", "DSOS254A", "DSOS404A", "DSOS604A", "DSOS804A", "MSOS054A", "MSOS104A", "MSOS204A", "MSOS254A", "MSOS404A", "MSOS604A", "MSOS804A", "DSAX96204Q", "DSOX96204Q", "DSAX95004Q", "DSOX95004Q", "DSAX93304Q", "DSOX93304Q", "DSAX92504Q", "DSOX92504Q", "DSAX92004Q", "DSOX92004Q"}
  T79 = typedef "cDAQ Session.ctl" = cluster{"mclk [Hz]":dbl, "ADC task":refnum<k21>, "mclk reference":string, "fs [Hz]":dbl, "queue adc cmd":refnum<queue>, "queue adc data":refnum<queue>, "adc proc ref":refnum<vi>, "channels":T80[], "last channels":T80[], "timeout":timestamp, "N":i32, "mclk mode":T81, "ext mclk source":tag}
  T80 = typedef "cDAQ Virtual Channel.ctl" = cluster{"Device":tag, "Channel id":i32, "btn clr":bool, "btn up":bool, "btn down":bool}
  T81 = typedef "cDAQ Master Clock Mode.ctl" = enum16{"Free running", "Export master clock", "Import master clock"}
  T82 = typedef "CMI ADS127L21 - Session.ctl" = cluster{"VISA":refnum<visa-resource-name>, "chn list":i32[], "record size":i32, "phys. channels":i32, "adc fifo size":i32, "channels":T83[], "ext refclk?":bool, "fs [Hz]":dbl, "ext refclk [Hz]":dbl, "meas refclk [Hz]":dbl, "EXTOUT mode":T87, "EXTOUT polarity":T88, "EXTOUT divisor":i32}
  T83 = typedef "CMI ADS127L21 - Record Channel.ctl" = cluster{"Range [Vpk]":T84, "Channel":i32, "Mode":T85, "Impedance":T86, "btn clr":bool, "btn up":bool, "btn down":bool}
  T84 = typedef "CMI ADS127L21 - Input Range.ctl" = dbl
  T85 = typedef "CMI ADS127L21 - Input Mode.ctl" = enum16{"Normal", "Inverted", "GND"}
  T86 = typedef "CMI ADS127L21 - Input Impedance.ctl" = enum16{"1M", "1k5"}
  T87 = typedef "CMI ADS127L21 - EXTOUT Mode.ctl" = enum16{"ADCCLK", "REFCLK", "SMPLCLK", "FIRST"}
  T88 = typedef "CMI ADS127L21 - EXTOUT Polarity.ctl" = enum16{"NORM", "INV"}
  T89 = typedef "Meas Sequence Item.ctl" = cluster{"config":T90, "data file path":path, "header file path":path, "group id":i32, "rec id":i32, "group done?":bool, "adc modified?":bool, "source modified?":bool, "progress [%]":dbl, "groups cnt":i32, "rec cnt":i32, "data file relative path":string, "meas root path":path, "calculate?":bool, "comment":string, "avg cnt":i32}
  T90 = typedef "Meas Sampling Configuration.ctl" = cluster{"count [smpl]":i64, "aperture [s]":dbl, "trigger":T32, "ranges [Vpk]":dbl[], "QWTB parameters":T91[], "sampling rate":T50}
  T91 = typedef "Meas Proc QWTB Algorithm Parameter Data.ctl" = cluster{"name":string, "numerics":dbl[], "strings":string[]}
  T92 = typedef "Meas Sequence Configuration.ctl" = cluster{"group setups":T90[], "rec count":i32, "range mode":T93, "fs mode":T94, "rng even":dbl, "rng odd":dbl, "folder":path, "name base":string, "meas id":i32, "settle [s]":dbl, "comment":string, "avg count":i32, "fs-abs-fr fr":dbl, "fs-abs-fr fs":dbl, "fs-div fr":dbl, "fs-div div":dbl, "fs-mn fr":dbl, "fs-mn mul":dbl, "fs-mn div":dbl, "fs-rat fr":dbl, "fs-rat rat":dbl}
  T93 = typedef "Meas Range Mode.ctl" = enum16{"Keep defaults", "Set All channels", "Set Odd and Even channels"}
  T94 = typedef "Meas Sampling Rate Mode.ctl" = enum16{"Frequency", "Period"}
  T95 = typedef "GOLPI Multi Process.lvlib/golpi_session_ref.ctl" = refnum<vi>
  T96 = typedef "Meas Process Config.ctl" = cluster{"mode":T97, "call after avgs?":bool, "calculate?":bool, "raw mode":T98, "QWTB":T100}
  T97 = typedef "Meas Process Mode.ctl" = enum16{"Raw", "QWTB"}
  T98 = typedef "Meas Process Raw Config.ctl" = cluster{"command":string, "result mode":T99, "res variable":string}
  T99 = typedef "Meas Process Raw Result Mode.ctl" = enum16{"Display console output (only Octave)", "Display string variable", "Display result file %respath%"}
  T100 = typedef "Meas Proc QWTB Setup.ctl" = cluster{"QWTB path":path, "alg filter path":string, "alg ids":string[], "alg parameters":string[], "parsed parameters":T91[], "selected alg id":string, "selected unc mode":T101, "qwtb mcc":i32, "qwtb timeout":i32, "qwtb covg":dbl, "qwtb ofs":i64, "qwtb lim data":i64, "multicore":T102, "unc once?":bool, "qwtb tstemp":T104, "octave reset":bool, "exec mode":T105}
  T101 = typedef "Meas Proc QWTB Uncertainty Mode.ctl" = enum16{"None", "GUF", "Monte Carlo"}
  T102 = typedef "Meas Proc QWTB Multicore Setup.ctl" = cluster{"jobs folder":path, "cores":i32, "max jobs":i32, "mode":T103}
  T103 = typedef "Meas Proc QWTB Multicore Type.ctl" = enum16{"Singlecore", "Multicore", "Multistation"}
  T104 = typedef "Meas Process Time Stamp Mode.ctl" = enum16{"Enabled (default)", "Disabled", "Relative to 1. record"}
  T105 = typedef "Meas Proc QWTB Exec Mode.ctl" = enum16{"Single-core", "Parallel Record Processing"}
  T106 = typedef "Corr Setup.ctl" = cluster{"transducers":cluster{"channels":T107[], "last path":path, "root path":path}, "digitizer":T108}
  T107 = typedef "Corr Tranducer Item.ctl" = cluster{"Path":path, "Ratio:":string, "Name:":string, "btn rem":bool, "btn up":bool, "btn down":bool, "s.n.:":string, "btn open":bool, "ratio o/i":dbl, "chn hi":u16, "chn lo":u16, "Phase index":i32, "btn edit":bool, "mpx chn":u16, "btn vdx1":bool, "btn csx1":bool, "invert":bool}
  T108 = typedef "Corr Digitizers.ctl" = cluster{"last path":path, "channel paths":path[], "channel idns":string[], "correction name":string, "channel names":string[], "folders to copy":path[], "channel valid":bool[], "correction path":path, "correction rel path":string, "rel folders to copy":string[], "root path":path}
  T109 = typedef "Assist Panel Setup.ctl" = cluster{"P":i32, "Q":i32, "rel shift":dbl, "ref freq":dbl, "min fs":dbl, "max fs tol":dbl, "min int":dbl, "max int":dbl, "max err":dbl, "max timeout":dbl}
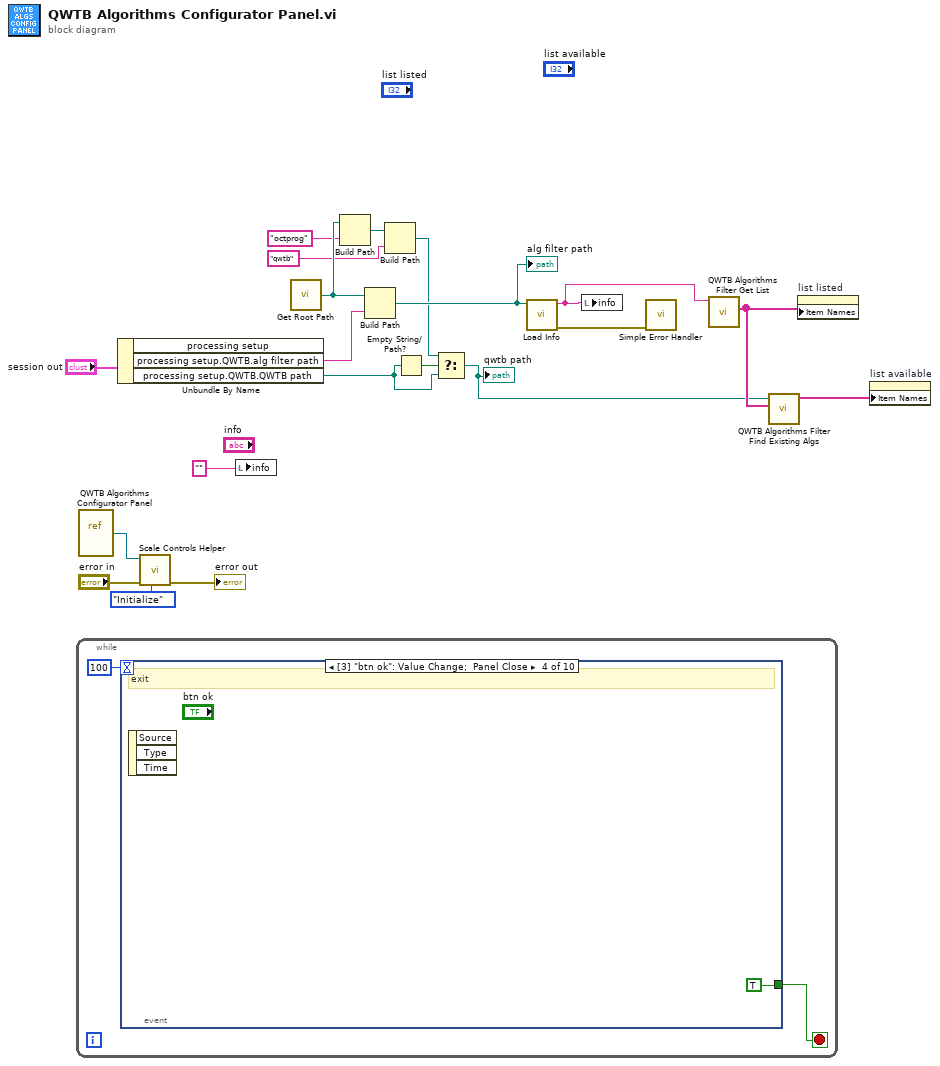
[diagram p0: block diagram]
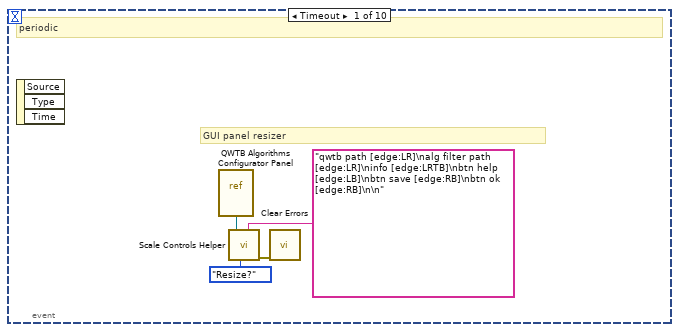
[diagram p2: hidden frame]
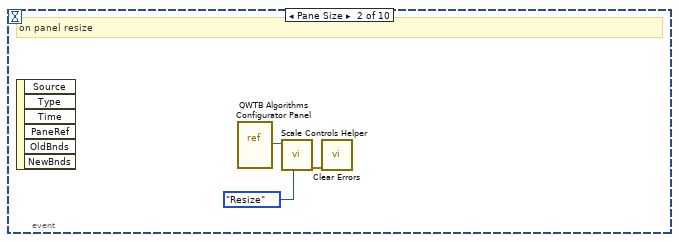
[diagram p3: hidden frame]
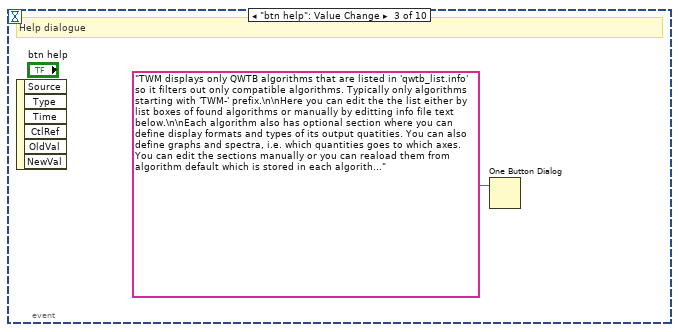
[diagram p4: hidden frame]
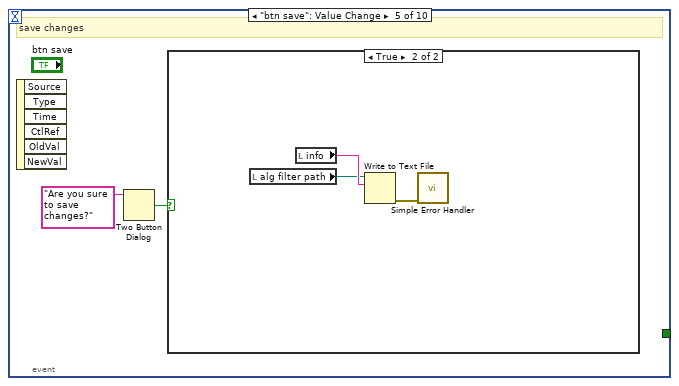
[diagram p5: hidden frame]
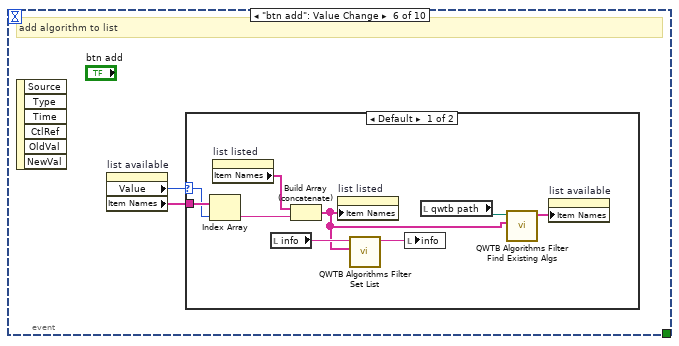
[diagram p7: hidden frame]
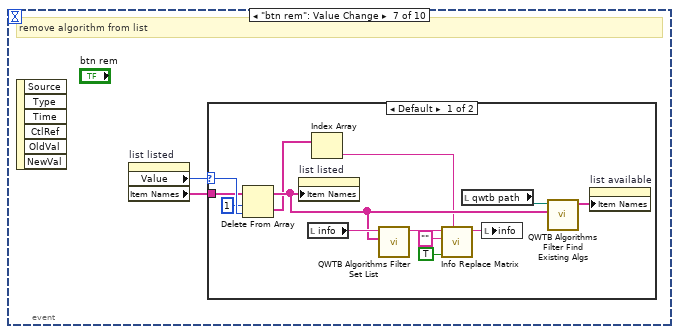
[diagram p9: hidden frame]
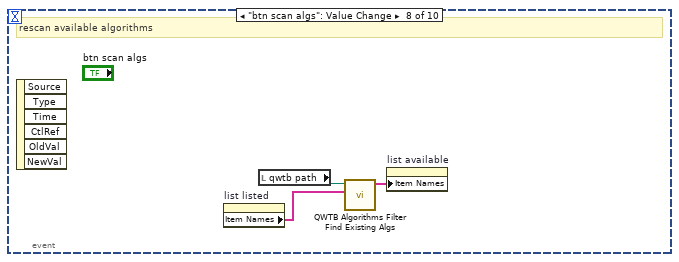
[diagram p11: hidden frame]
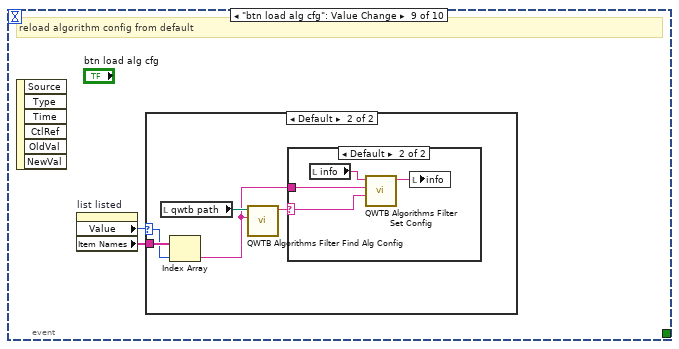
[diagram p12: hidden frame]
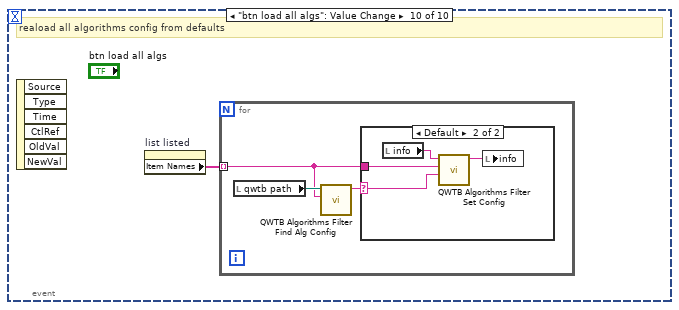
[diagram p15: hidden frame]
diagram:
  n1 = while {
    stop <- w22 stop-if-true
    n2 = event shown="[3] \"btn ok\": Value Change;  Panel Close" {
      selector: _ -> [_ _ _ _ _ _ _ _ _ _]
      dyn-events: _ -> [_ _ _ _ _ _ _ _ _ _]
      timeout: 100 -> [_ _ _ _ _ _ _ _ _ _]
      tunnel: [_ _ _ TRUE _ _ _ _ _ _] -> w22
      event Timeout {
        # "GUI panel resizer"
        # "periodic"
        n3 = event-data() -> ()  [unwired: 1 in, 3 out]
        n4 = vi-ref "QWTB Algorithms Configurator Panel.vi"() -> (w26:refnum<vi>)
        n5 = call "Scale Controls Helper.vi"("rules"="qwtb path [edge:LR]\nalg filter path [edge:LR]\ninfo [edge:LRTB]\nbtn help [edge:LB]\nbtn save [edge:RB]\nbtn ok [edge:RB]\n\n", "Action (Initialize)"=enum16{"Initialize", "Resize", "Resize?"}."Resize?", "vi reference"=w26) -> ("error out"=w23:errorcluster)  [unwired: 8 in]
        n6 = call <vilib>:"Clear Errors.vi"("error in (no error)"=w23) -> ()  [unwired: 5 in, 2 out]
      }
      event Pane Size {
        # "on panel resize"
        n7 = event-data() -> ()  [unwired: 1 in, 6 out]
        n8 = vi-ref "QWTB Algorithms Configurator Panel.vi"() -> (w29:refnum<vi>)
        n9 = call "Scale Controls Helper.vi"("Action (Initialize)"=enum16{"Initialize", "Resize", "Resize?"}."Resize", "vi reference"=w29) -> ("error out"=w28:errorcluster)  [unwired: 9 in]
        n10 = call <vilib>:"Clear Errors.vi"("error in (no error)"=w28) -> ()  [unwired: 5 in, 2 out]
      }
      event "btn help": Value Change {
        # "Help dialogue"
        n11 = event-data() -> ()  [unwired: 1 in, 6 out]
        n12 = One Button Dialog(message="TWM displays only QWTB algorithms that are listed in 'qwtb_list.info' so it filters out only compatible algorithms. Typically only algorithms starting with 'TWM-' prefix.\n\nHere you can edit the the list either by list boxes of found algorithms or manually by editting info file text below.\n\nEach algorithm also has optional section where you can define display formats and types of its output quatities. You can also define graphs and spectra, i.e. which quantities goes to which axes. You can edit the sections manually or you can reaload them from algorithm default which is stored in each algorithm's folder in file 'alg_twm.info'.") -> ()  [unwired: 1 in, 1 out]
      }
      event "btn ok": Value Change; Panel Close {
        # "exit"
        n13 = event-data() -> ()  [unwired: 1 in, 3 out]
      }
      event "btn save": Value Change {
        # "save changes"
        n14 = event-data() -> ()  [unwired: 1 in, 6 out]
        n15 = Two Button Dialog(message="Are you sure to save changes?") -> (T button?=w33:bool)  [unwired: 2 in]
        n16 = case shown="True" w33 {
          frame False {
          }
          frame True {
            n17 = local read "alg filter path"() -> (w34:path)
            n18 = local read "info"() -> (w36:string)
            n19 = Write to Text File(file (use dialog)=w34, text=w36) -> (error out=w35:errorcluster)  [unwired: 2 in, 2 out]
            n20 = call <vilib>:"Simple Error Handler.vi"("error in (no error)"=w35) -> ()  [unwired: 4 in, 5 out]
          }
        }
      }
      event "btn add": Value Change {
        # "add algorithm to list"
        n21 = event-data() -> ()  [unwired: 1 in, 6 out]
        n22 = property on="list available" class="LstBox (strict)"() -> ("Value"=w38:i32, "Item Names"=w37:string[])  [unwired: 2 in, 2 out]
        n23 = case shown="Default" w38 {
          selector: w38 -> [w46 _]
          tunnel: w37 -> [w47 _]
          frame Default {
            n24 = Index Array(array=w47, index=w46) -> (element=w44:string)
            n25 = property on="list listed" class="LstBox (strict)"() -> ("Item Names"=w45:string[])  [unwired: 2 in, 2 out]
            n26 = local read "info"() -> (w42:string)
            n27 = Build Array (concatenate)(w45, w44) -> (w39:string[])
            n28 = property on="list listed" class="LstBox (strict)"("Item Names"=w39) -> ()  [unwired: 2 in, 2 out]
            n29 = call "QWTB Algorithms Filter Set List.vi"("algs list"=w39, "info data"=w42) -> ("info data out"=w43:string)  [unwired: 9 in]
            n30 = local write "info"(w43) -> ()
            n31 = local read "qwtb path"() -> (w41:path)
            n32 = call "QWTB Algorithms Filter Find Existing Algs.vi"("exclude algs list"=w39, "QWTB path"=w41) -> ("available algs list"=w40:string[])  [unwired: 9 in]
            n33 = property on="list available" class="LstBox (strict)"("Item Names"=w40) -> ()  [unwired: 2 in, 2 out]
          }
          frame -1 {
          }
        }
      }
      event "btn rem": Value Change {
        # "remove algorithm from list"
        n34 = event-data() -> ()  [unwired: 1 in, 6 out]
        n35 = property on="list listed" class="LstBox (strict)"() -> ("Value"=w49:i32, "Item Names"=w48:string[])  [unwired: 2 in, 2 out]
        n36 = case shown="Default" w49 {
          selector: w49 -> [w58 _]
          tunnel: w48 -> [w54 _]
          frame Default {
            n37 = Delete From Array(array=w54, length=1, index=w58) -> (deleted portion=w53:string[], array with subset deleted=w60:string[])
            n38 = property on="list listed" class="LstBox (strict)"("Item Names"=w60) -> ()  [unwired: 2 in, 2 out]
            n39 = local read "info"() -> (w62:string)
            n40 = Index Array(array=w53) -> (element=w52:string)  [unwired: 1 in]
            n41 = call "QWTB Algorithms Filter Set List.vi"("algs list"=w60, "info data"=w62) -> ("info data out"=w56:string)  [unwired: 9 in]
            n42 = call "Info Replace Matrix.vi"("key description to replace"=w52, "Is Section (False)"=TRUE, "info data to paste"="", "info data in"=w56) -> ("info data out"=w55:string)  [unwired: 7 in]
            n43 = local read "qwtb path"() -> (w61:path)
            n44 = local write "info"(w55) -> ()
            n45 = call "QWTB Algorithms Filter Find Existing Algs.vi"("exclude algs list"=w60, "QWTB path"=w61) -> ("available algs list"=w59:string[])  [unwired: 9 in]
            n46 = property on="list available" class="LstBox (strict)"("Item Names"=w59) -> ()  [unwired: 2 in, 2 out]
          }
          frame -1 {
          }
        }
      }
      event "btn scan algs": Value Change {
        # "rescan available algorithms"
        n47 = event-data() -> ()  [unwired: 1 in, 6 out]
        n48 = property on="list listed" class="LstBox (strict)"() -> ("Item Names"=w63:string[])  [unwired: 2 in, 2 out]
        n49 = local read "qwtb path"() -> (w65:path)
        n50 = call "QWTB Algorithms Filter Find Existing Algs.vi"("exclude algs list"=w63, "QWTB path"=w65) -> ("available algs list"=w64:string[])  [unwired: 9 in]
        n51 = property on="list available" class="LstBox (strict)"("Item Names"=w64) -> ()  [unwired: 2 in, 2 out]
      }
      event "btn load alg cfg": Value Change {
        # "reload algorithm config from default"
        n52 = event-data() -> ()  [unwired: 1 in, 6 out]
        n53 = property on="list listed" class="LstBox (strict)"() -> ("Value"=w67:i32, "Item Names"=w66:string[])  [unwired: 2 in, 2 out]
        n54 = case shown="Default" w67 {
          selector: w67 -> [_ w69]
          tunnel: w66 -> [_ w70]
          frame -1 {
          }
          frame Default {
            n55 = local read "qwtb path"() -> (w72:path)
            n56 = Index Array(array=w70, index=w69) -> (element=w68:string)
            n57 = call "QWTB Algorithms Filter Find Alg Config.vi"("algorithm name"=w68, "QWTB path"=w72) -> ("section part"=w71:string)  [unwired: 9 in]
            n58 = case shown="Default" w71 {
              selector: w71 -> [_ w75]
              tunnel: w68 -> [_ w76]
              frame "" {
              }
              frame Default {
                n59 = local read "info"() -> (w73:string)
                n60 = call "QWTB Algorithms Filter Set Config.vi"("new algorithm config section data"=w75, "algorithm name"=w76, "info data"=w73) -> ("info data out"=w74:string)  [unwired: 8 in]
                n61 = local write "info"(w74) -> ()
              }
            }
          }
        }
      }
      event "btn load all algs": Value Change {
        # "reaload all algorithms config from defaults"
        n62 = event-data() -> ()  [unwired: 1 in, 6 out]
        n63 = property on="list listed" class="LstBox (strict)"() -> ("Item Names"=w77:string[])  [unwired: 2 in, 2 out]
        n64 = for {
          tunnel: w77 -> [w78] mode=indexing
          n65 = local read "qwtb path"() -> (w80:path)
          n66 = call "QWTB Algorithms Filter Find Alg Config.vi"("algorithm name"=w78, "QWTB path"=w80) -> ("section part"=w79:string)  [unwired: 9 in]
          n67 = case shown="Default" w79 {
            selector: w79 -> [_ w83]
            tunnel: w78 -> [_ w84]
            frame "" {
            }
            frame Default {
              n68 = local read "info"() -> (w81:string)
              n69 = call "QWTB Algorithms Filter Set Config.vi"("new algorithm config section data"=w83, "algorithm name"=w84, "info data"=w81) -> ("info data out"=w82:string)  [unwired: 8 in]
              n70 = local write "info"(w82) -> ()
            }
          }
        }
      }
    }
  }
  n71 = vi-ref "QWTB Algorithms Configurator Panel.vi"() -> (w4:refnum<vi>)
  n72 = Unbundle By Name("session out") -> ("processing setup.QWTB.alg filter path"=w10:string, "processing setup.QWTB.QWTB path"=w7:path)  [unwired: 1 out]
  n73 = call "Scale Controls Helper.vi"("Action (Initialize)"=enum16{"Initialize", "Resize", "Resize?"}."Initialize", "error in (no error)"="error in", "vi reference"=w4) -> ("error out"=→"error out":errorcluster)  [unwired: 8 in]
  n74 = local write "info"("" ("Content")) -> ()
  n75 = call "Get Root Path.vi"() -> ("root path"=w14:path)
  n76 = Build Path(base path=w14, name or relative path="octprog") -> (appended path=w12:path)
  n77 = Build Path(base path=w14, name or relative path=w10) -> (appended path=w9:path)
  "alg filter path" <- w9
  n78 = Build Path(base path=w12, name or relative path="qwtb") -> (appended path=w6:path)
  n79 = Empty String/Path?(string/path=w7) -> (empty?=w8:bool)
  n80 = Select(t=w6, s=w8, f=w7) -> (s? t:f=w5:path)
  "qwtb path" <- w5
  n81 = call "Load Info.vi"("filename"=w9) -> ("error out"=w17:errorcluster, "info data"=w16:string)  [unwired: 9 in]
  n82 = local write "info"(w16) -> ()
  n83 = call <vilib>:"Simple Error Handler.vi"("error in (no error)"=w17) -> ()  [unwired: 4 in, 5 out]
  n84 = call "QWTB Algorithms Filter Get List.vi"("info data"=w16) -> ("algs list"=w15:string[])  [unwired: 9 in, 1 out]
  n85 = call "QWTB Algorithms Filter Find Existing Algs.vi"("exclude algs list"=w15, "QWTB path"=w5) -> ("available algs list"=w18:string[])  [unwired: 9 in]
  n86 = property on="list listed" class="LstBox (strict)"("Item Names"=w15) -> ()  [unwired: 2 in, 2 out]
  n87 = property on="list available" class="LstBox (strict)"("Item Names"=w18) -> ()  [unwired: 2 in, 2 out]
